vi "Distance Drive Checker.vi"(9 "Current Heading Target":dbl, 10 "Current Y Target":dbl, 11 "Current X Target":dbl) -> (3 "Distance Drive Done?":bool)   [LabVIEW 2014]
uses:
  Robot Global Data.vi
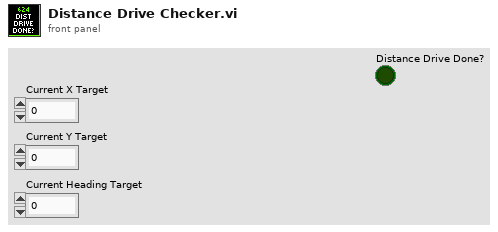
[diagram p1: front panel]
types:
  T1 = typedef "Drivetrain Status.ctl" = cluster{"Y (Throttle)":dbl, "X (Steer)":dbl, "Translation X":dbl, "Center Wheel Down":bool, "Mode":T2, "Distance Drive finished?":bool, "Y Target":dbl, "X Target":dbl, "Heading Target":dbl}
  T2 = typedef "Drivetrain Mode.ctl" = enum16{"Manual", "Gyro Steer", "Vision Steer", "Drive Distance"}
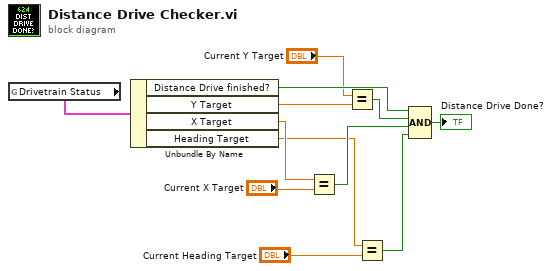
[diagram p0: block diagram]
diagram:
  n1 = global read "Robot Global Data.vi" "Drivetrain Status"() -> (w12:T1)
  n2 = Unbundle By Name(w12) -> ("Distance Drive finished?"=w11:bool, "Y Target"=w9:dbl, "X Target"=w6:dbl, "Heading Target"=w4:dbl)
  n3 = Equal?(x=w6, y="Current X Target") -> (x = y?=w5:bool)
  n4 = Equal?(x="Current Y Target", y=w9) -> (x = y?=w8:bool)
  n5 = Equal?(x=w4, y="Current Heading Target") -> (x = y?=w2:bool)
  n6 = Compound Arithmetic op=AND(w11, w8, w5, w2) -> (→"Distance Drive Done?":bool)
